vi "X2 Encoder Count.vi"(4 "phase B_prev":bool, 5 "phase A":bool, 6 "phase B":bool, 7 "phase A_prev":bool, 11 "count in":i32) -> (2 "count changed?":bool, 3 "count out":i32)   [LabVIEW 2017, in "NI_Robotics Utilities.lvlib"]
uses:
  <vilib>/robotics/Utilities/NI_Robotics Utilities.lvlib
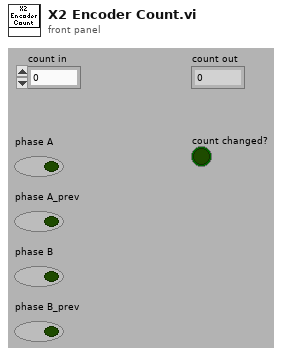
[diagram p1: front panel]
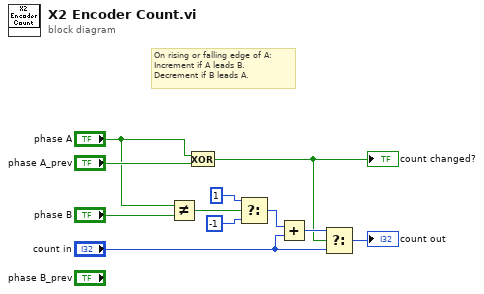
[diagram p0: block diagram]
diagram:
  # "On rising or falling edge of A:\nIncrement if A leads B.\nDecrement if B leads A."
  n1 = Not Equal?(x="phase A", y="phase B") -> (x != y?=w1:bool)
  n2 = Exclusive Or(1:"phase A_prev", 2:"phase A") -> (0:w4:bool)
  "count changed?" <- w4
  n3 = Select(t=1 ("count in"), s=w1, f=-1 ("count in")) -> (s? t:f=w6:i32)
  n4 = Add(x=w6, y="count in") -> (x+y=w5:i32)
  n5 = Select(t=w5, s=w4, f="count in") -> (s? t:f=→"count out":i32)
